vi "filterWheel.vi"(8 "serial  port":i32, 10 "position":i32) -> ()   [LabVIEW 2013]
panel:
  in  "error in":T1
  out "error out":T1
  out "Timeout (3s)":i32
  out "Baud (115200)":i32
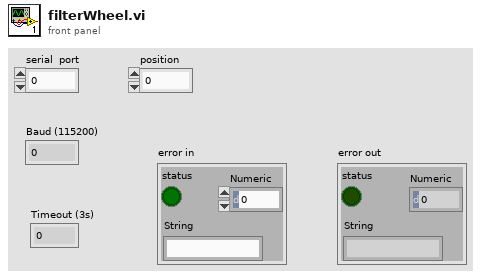
[diagram p1: front panel]
types:
  T1 = cluster{"status":bool, "Numeric":i32, "String":string}
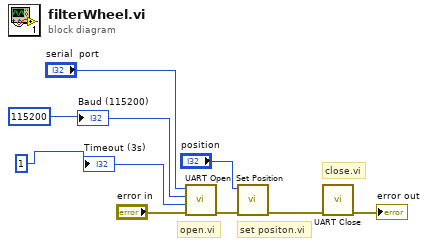
[diagram p0: block diagram]
diagram:
  w1 = 1 ("Timeout (3s)")
  w2 = 115200 ("Baud (115200)")
  # "set positon.vi"
  # "open.vi"
  # "close.vi"
  n1 = call "UART Open.vi"("error in (no error)"="error in", "Timeout (3s)"=w1, "Baud (115200)"=w2, "Serial Port"="serial  port") -> ("error out"=w4:errorcluster)  [unwired: 6 in, 1 out]
  n2 = call "Set Position.vi"("error in (no error)"=w4, "Position"="position") -> ("error out"=w3:errorcluster)  [unwired: 9 in]
  n3 = call "UART Close.vi"("error in (no error)"=w3) -> ("error out"=→"error out":errorcluster)  [unwired: 10 in]
  "Baud (115200)" <- w2
  "Timeout (3s)" <- w1
